vi "Get Double Complex.vi"(7 "data type of variable":cdb, 8 "error in":errorcluster, 10 "variable name":string, 11 "GOLPI ref. in":T1={"pipe handle"={"lv_proc.dll file path"=path "", "process instance handle"=[], "debug mode"=FALSE, "debug data"=[]}, "fast read timeout [ms]"=500, "fast read settle time [ms]"=10, "fast read to multiple [ms]"=1, "max elements per input line"=100, "slow read timeout [ms]"=5000, "stdin double format specifier"="%_16e", "max elements per stdout output column"=100, "console mode bitstream"=FALSE, "bitstream first read timeout [ms]"=1000, "bitstream read timeout [ms]"=50, "struct transfer possible"=FALSE, "matlab mode"=FALSE}) -> (0 "error out":errorcluster, 2 "value":cdb format="%.2f", 3 "GOLPI ref. out":T1={"pipe handle"={"lv_proc.dll file path"=path "", "process instance handle"=[], "debug mode"=FALSE, "debug data"=[]}, "fast read timeout [ms]"=500, "fast read settle time [ms]"=10, "fast read to multiple [ms]"=1, "max elements per input line"=100, "slow read timeout [ms]"=5000, "stdin double format specifier"="%_16e", "max elements per stdout output column"=100, "console mode bitstream"=FALSE, "bitstream first read timeout [ms]"=1000, "bitstream read timeout [ms]"=50, "struct transfer possible"=FALSE, "matlab mode"=FALSE})   [LabVIEW 2020, in "GOLPI library.lvlib"]
doc: "Part of polymorph Get Variable.vi"
uses:
  GOLPI library.lvlib
  GOLPI reference Type Def.ctl
  Pipe Handle.ctl
  Custom Error Codes Enum Type Def.vi
  Bitstream Data Type.ctl
  LV Process library.lvlib
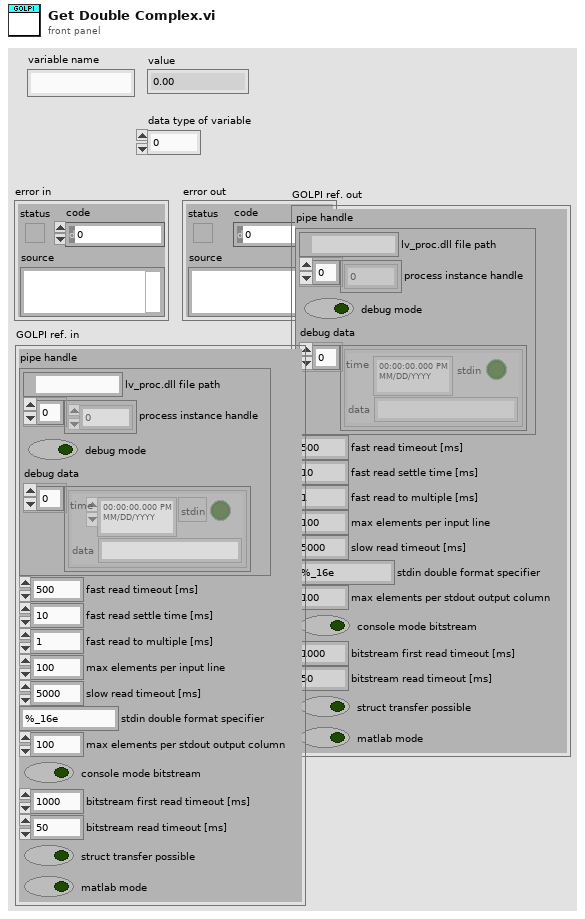
[diagram p1: front panel]
types:
  T1 = typedef "GOLPI library.lvlib/GOLPI reference Type Def.ctl" = cluster{"pipe handle":T2, "fast read timeout [ms]":u32, "fast read settle time [ms]":u32, "fast read to multiple [ms]":u32, "max elements per input line":u32, "slow read timeout [ms]":u32, "stdin double format specifier":string, "max elements per stdout output column":u32, "console mode bitstream":bool, "bitstream first read timeout [ms]":u32, "bitstream read timeout [ms]":u32, "struct transfer possible":bool, "matlab mode":bool}
  T2 = typedef "LV Process library.lvlib/Pipe Handle.ctl" = cluster{"lv_proc.dll file path":path, "process instance handle":u32[], "debug mode":bool, "debug data":cluster{"time":timestamp, "stdin":bool, "data":string}[]}
  T3 = typedef "GOLPI library.lvlib/Custom Error Codes Enum Type Def.vi" = enum16{"no error", "00 working directory PAR1 missing", "01 octave binary PAR1 missing", "02 octave report error PAR1", "03 empty output last cmd PAR1", "04 missing temporary file PAR1", "05 pwd PAR 1 not exist", "06 oct package not installed", "07 octave default binary missing", "10 var PAR1 not string, vect", "11 var PAR1 not num, scal, ~compl", "12 var PAR1 not num, scal, compl", "13 var PAR1 not num, vect, ~compl", "14 var PAR1 not num, vect, compl", "15 var PAR1 not num, mat, ~compl", "16 var PAR1 not num, mat, ~compl", "30 read timeout", "60 bitstream transport failed", "61 bitstream decode error PAR1", "62 bitstream cannot be set", "70 struct transfer not possible", "80 struct: cluster elem. PAR1 not implem.", "81 struct: structure field PAR1 not implem.", "82 struct: size mismatch of PAR1", "83 struct: type mismatch of PAR1", "98 internal error", "99 not finished", "90 Not supported in Matlab mode", "91 Matlab variable transfer error", "92 Matlab Script Error"}
  T4 = typedef "GOLPI library.lvlib/Bitstream Data Type.ctl" = enum16{"dummy", "int", "uint", "float", "complex", "str", "real numeric"}
  T5 = typedef "GOLPI library.lvlib/Bitstream Data.ctl" = cluster{"double":dbl[][], "cplx double":cdb[][], "int64":i64[][], "uint64":u64[][], "str":string[], "data type":T4}
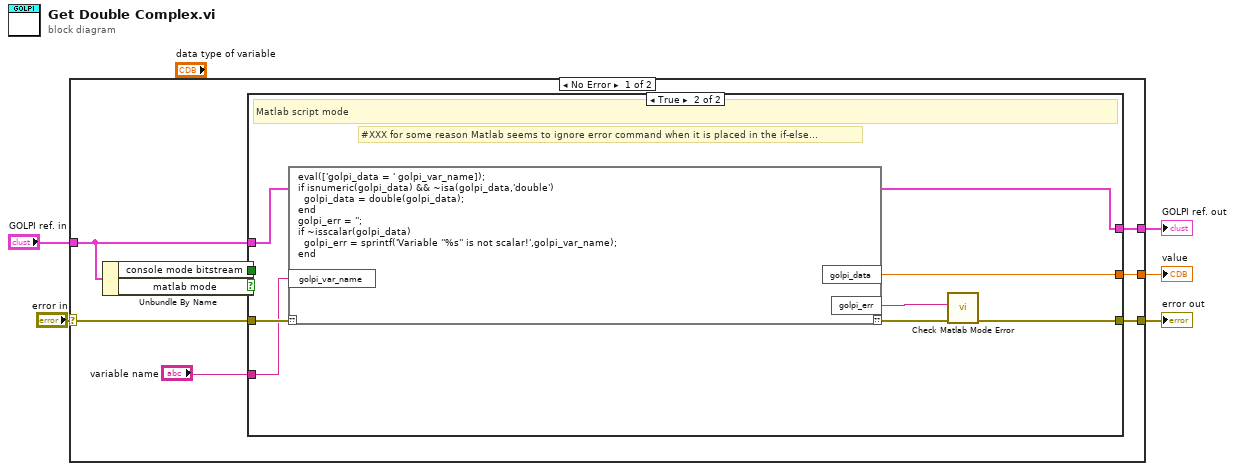
[diagram p0: block diagram]
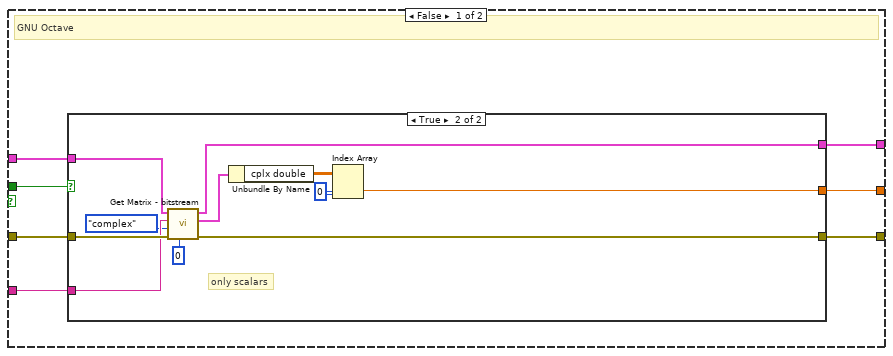
[diagram p2: hidden frame]
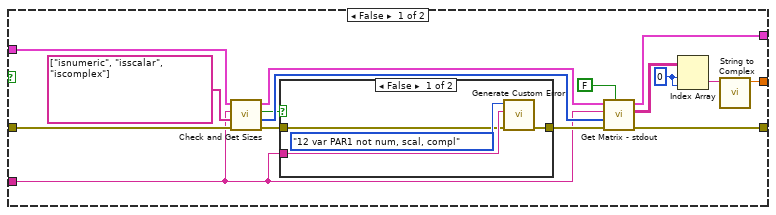
[diagram p3: hidden frame]
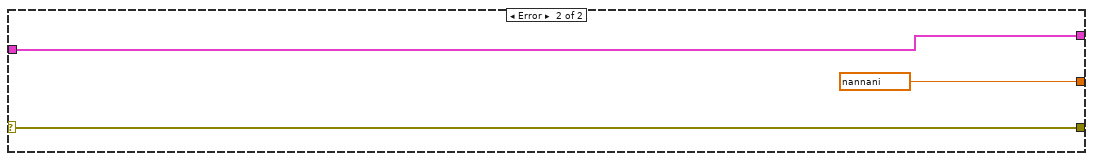
[diagram p5: hidden frame]
diagram:
  n1 = case shown="No Error" "error in" {
    selector: "error in" -> [w13 w62]
    tunnel: [w10 cdb nan+nani ("t")] -> w5
    tunnel: [w12 w62] -> w4
    tunnel: "GOLPI ref. in" -> [w9 w60]
    tunnel: [w11 w60] -> w1
    frame No Error {
      n2 = Unbundle By Name(w9) -> ("console mode bitstream"=w8:bool, "matlab mode"=w6:bool)
      n3 = case shown="True" w6 {
        tunnel: w13 -> [w20 w59]
        tunnel: [w19 w53] -> w12
        tunnel: [w18 w58] -> w11
        tunnel: [w17 w56] -> w10
        tunnel: w9 -> [w16 w58]
        tunnel: w8 -> [w15 _]
        tunnel: "variable name" -> [w14 w57]
        frame False {
          # "GNU Octave"
          n4 = case shown="True" w15 {
            tunnel: w20 -> [w35 w52]
            tunnel: [w32 w43] -> w19
            tunnel: [w25 w47] -> w18
            tunnel: [w23 w44] -> w17
            tunnel: w16 -> [w22 w51]
            tunnel: w14 -> [w21 w50]
            frame False {
              w29 = 0 ("index (row)")
              n5 = call "Check and Get Sizes.vi"("error in (no error)"=w35, "test commands"=string[] ["isnumeric", "isscalar", "iscomplex"], "variable name"=w21, "GOLPI ref. in"=w22) -> ("error out"=w36:errorcluster, "octave sizes"=w31:i32[], "all tests OK?"=w30:bool, "GOLPI ref. out"=w26:T1)  [unwired: 4 in]
              n6 = case shown="False" w30 {
                tunnel: [w37 w41] -> w33
                tunnel: w36 -> [w38 w41]
                tunnel: w21 -> [w39 _]
                frame False {
                  n7 = call "Generate Custom Error.vi"("error in"=w38, "PAR1"=w39, "GOLPI error"=Custom_Error_Codes_Enum_Type_Def.vi."12 var PAR1 not num, scal, compl" ("Enum")) -> ("error out"=w37:errorcluster)  [unwired: 8 in]
                }
                frame True {
                }
              }
              n8 = call "Get Matrix - stdout.vi"("is string?"=FALSE ("is string"), "error in (no error)"=w33, "octave sizes"=w31, "variable name"=w21, "GOLPI ref. in"=w26) -> ("error out"=w32:errorcluster, "array"=w28:string[][], "GOLPI ref. out"=w25:T1)  [unwired: 4 in]
              n9 = Index Array(array=w28, index (row)=w29, index (col)=w29) -> (element=w27:string)
              n10 = call "String to Complex.vi"("string"=w27) -> ("complex number"=w23:cdb)  [unwired: 10 in]
            }
            frame True {
              w42 = 0 ("index (row)")
              # "only scalars"
              n11 = call "Get Matrix - bitstream.vi"("max dimensions (0: scalar)"=0, "error in (no error)"=w52, "data type"=Bitstream_Data_Type."complex", "variable name"=w50, "GOLPI ref. in"=w51) -> ("error out"=w43:errorcluster, "data"=w46:T5, "GOLPI ref. out"=w47:T1)  [unwired: 4 in]
              n12 = Unbundle By Name(w46) -> ("cplx double"=w45:cdb[][])
              n13 = Index Array(array=w45, index (row)=w42, index (col)=w42) -> (element=w44:cdb)
            }
          }
        }
        frame True {
          # "#XXX for some reason Matlab seems to ignore error command when it is placed in the if-else..."
          # "Matlab script mode"
          n14 = script code="eval(['golpi_data = ' golpi_var_name]);\nif isnumeric(golpi_data) && ~isa(golpi_data,'double')\n  golpi_data = double(golpi_data);\nend\ngolpi_err = '';\nif ~isscalar(golpi_data)\n  golpi_err = sprintf('Variable ''%s'' is not scalar!',golpi_var_name);\nend"("??"=w59, "golpi_var_name"=w57) -> ("??"=w55:errorcluster, "golpi_data"=w56:cdb, "golpi_err"=w54:string)
          n15 = call "Check Matlab Mode Error.vi"("error in"=w55, "custom error string (empty)"=w54) -> ("error out"=w53:errorcluster)  [unwired: 9 in]
        }
      }
    }
    frame Error {
    }
  }
  "value" <- w5
  "error out" <- w4
  "GOLPI ref. out" <- w1
